vi "testoct.vi"() -> ()   [LabVIEW 2020]
uses:
  Utilities/Calculation related/Globals for GOLPI.vi
  external libraries/GOLPI 0.7.3.1 source distribution LV 20.0 32 bit/GOLPI library.lvlib
panel:
  in  "GNU Octave path":path
  out "error out":errorcluster
  in  "Stop":bool
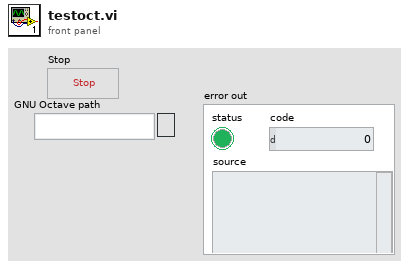
[diagram p1: front panel]
types:
  T1 = typedef "Type definitions to be saved.ctl" = cluster{"Common properties":T2, "AC Source":T3, "DC meter":T5, "CE measurement":T7, "FR measurement":T8, "FR template":T9, "CE template":T10, "PJVS":T11, "SS measurement":T15}
  T2 = typedef "Common properties.ctl" = cluster{"Measurement status ref":refnum<vi>, "TWM Status ref":refnum<vi>, "Abort ref":refnum<vi>, "Skip waiting ref":refnum<vi>, "GNU Octave path":path, "TWM+QWTB path":path, "lvlib path":path, "TWM pipe":string, "PJVS status ref":refnum<vi>, "WAC path":path}
  T3 = typedef "AC Source.ctl" = cluster{"AC Source type":T4, "VISA":refnum<visa-resource-name>, "Ref. clock (Hz)":dbl, "status ref":refnum<vi>}
  T4 = typedef "AC Source type.ctl" = enum16{"Fluke 5XXX calibrator", "Tektronix AFG3000 series", "dummy", "Agilent 331xxA to 332xxA", "Agilent 335xxA to 336xxA"}
  T5 = typedef "DC meter.ctl" = cluster{"DC meter type":T6, "DC meter VISA":refnum<visa-resource-name>, "NPLC":dbl, "status ref":refnum<vi>}
  T6 = typedef "DC meter type.ctl" = enum16{"H/A/K 3458", "Fluke 8508A", "dummy", "Keithley 2182"}
  T7 = typedef "CE measurement.ctl" = cluster{"Signal frequencies (Hz)":dbl[], "Signal amplitudes (V)":dbl[], "Sampling frequencies (Hz)":dbl[], "Record lengths (multiples of periods)":dbl[], "TWM data root directory":path, "TWM mreasurements directories":path[], "Calculate RMS from samples":bool, "RMS algorithm":string, "Settle down after AC source change (s)":dbl, "Skip PJVS setup":bool, "Measurement template file":path, "Row of START keyword":i32, "Row of STOP keyword":i32, "Measurement template line":i32[], "Switch position":dbl[], "FR fit mat file":path, "Recalculate-skip already calculated":bool}
  T8 = typedef "FR measuement.ctl" = cluster{"Measurement frequencies (Hz)":dbl[], "Sampling frequency (Hz)":dbl, "Signal amplitude (V)":dbl, "AC-DC settle time (s)":dbl, "Record length (multiples of period)":dbl[], "Measurement template file":path, "Row of START keyword":i32, "Row of STOP keyword":i32, "Calculate RMS from samples":bool, "AC-DC warm up time (s)":dbl, "Measurement template line":i32[], "DC meter readings No.":i32, "Algorithm":string, "Simultaneous measurement":bool, "Recalculate-skip already calculated":bool}
  T9 = typedef "FR template.ctl" = cluster{"Keywords column":i32, "Sig. freq. column":i32, "Rec. len. column":i32, "Meas. points. row min to read":i32, "Meas. points. row max to read":i32, "Properties column":i32, "Properties row start":i32, "Properties row end":i32, "Keyword START regexp":string, "Keyword STOP regexp":string, "HW data column":i32, "HW data row start":i32, "HW data row end":i32, "TIme and date column start":i32, "Digitizer value column start ":i32, "DC mean column start ":i32, "DC readings column start":i32}
  T10 = typedef "CE template.ctl" = cluster{"Keywords column":i32, "Sig. freq. column":i32, "Rec. len. column":i32, "Switch pos column":i32, "Meas. points. row min to read":i32, "Meas. points. row max to read":i32, "Properties column":i32, "Properties row start":i32, "Properties row end":i32, "Keyword START regexp":string, "Keyword STOP regexp":string, "HW data column":i32, "HW data row start":i32, "HW data row end":i32, "TIme and date column start":i32, "Digitizer value column start ":i32}
  T11 = typedef "PJVS.ctl" = cluster{"PJVS type":T12, "Status Refnum":refnum<vi>, "AC-supraVOLTcontrol":cluster{"IP address:port (0.0.0.0:0000)":string, "Timeouts":T13, "Simulation mode":bool, "Debug mode":bool}, "NPL bias source":cluster{"DataSocketCluster":T14}, "Manual PJVS":cluster{"PJVS frequency (Hz)":dbl, "Reference voltages (V)":dbl[], "File with PJVS voltages":path}, "VTT PJVS":cluster{"some VTT only property":string}}
  T12 = typedef "PJVS Type.ctl" = enum16{"AC-supraVOLTcontrol", "JV modified NPL bias control", "Manual PJVS", "VTT PJVS"}
  T13 = typedef "ACSVcontrol-driver.lvlib/Timeouts.ctl" = cluster{"TCP Read & Write (ms)":i32, "Sensors readout":i32, "PJVS setup":i32, "Nullmeter readout":i32, "Multiplexer setup":i32, "57XX setup":i32, "Generator setup":i32, "Synthesizer setup":i32, "Sampler readout":i32}
  T14 = typedef "DataSocketCluster external.ctl" = cluster{"Server Machine":string, "Client Machine":string, "Data":string, "TimeStamp":dbl, "Count":i32, "Target Process":string}
  T15 = typedef "SS measurement.ctl" = cluster{"Signal frequencies (Hz)":dbl[], "Signal amplitudes (V)":dbl[], "Sampling frequencies (Hz)":dbl[], "Record lengths (multiples of periods)":dbl[], "Calculate results":bool, "Algorithm":string, "TWM data directories":path[], "Settle down after AC source change (s)":dbl, "PJVS frequencies (Hz)":dbl[], "PJVS reference voltages":dbl[][], "Requested PJVS steps":u32[], "FR fit path":path, "Measure CE":bool, "Measure CE before":bool, "Measure CE after":bool, "CE fit path":path, "Measure digitizer gain":bool, "Measure digitizer gain before":bool, "Measure digitizer gain after":bool, "Digitizer gain":dbl}
  T16 = typedef "GOLPI library.lvlib/GOLPI reference Type Def.ctl" = cluster{"pipe handle":T17, "fast read timeout [ms]":u32, "fast read settle time [ms]":u32, "fast read to multiple [ms]":u32, "max elements per input line":u32, "slow read timeout [ms]":u32, "stdin double format specifier":string, "max elements per stdout output column":u32, "console mode bitstream":bool, "bitstream first read timeout [ms]":u32, "bitstream read timeout [ms]":u32, "struct transfer possible":bool, "matlab mode":bool}
  T17 = typedef "LV Process library.lvlib/Pipe Handle.ctl" = cluster{"lv_proc.dll file path":path, "process instance handle":u32[], "debug mode":bool, "debug data":cluster{"time":timestamp, "stdin":bool, "data":string}[]}
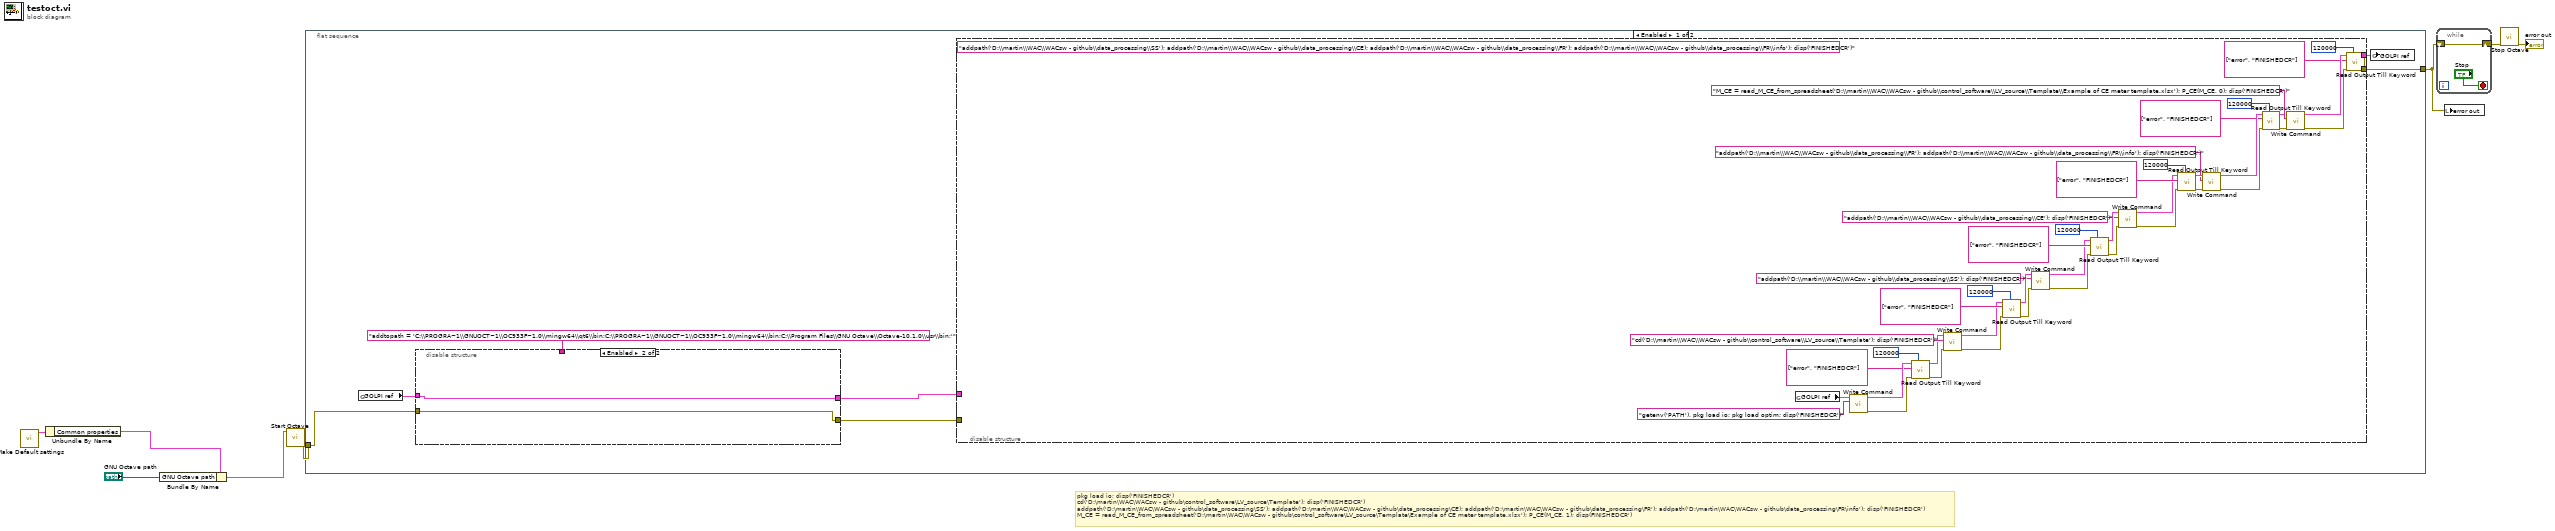
[diagram p0: block diagram]
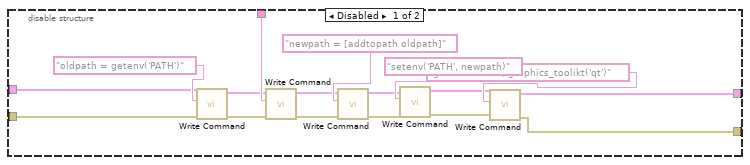
[diagram p2: hidden frame]
diagram:
  # "pkg load io; disp('FINISHEDCR')\ncd('D:\\martin\\WAC\\WACsw - github\\control_software\\LV_source\\Template'); disp('FINISHEDCR')\naddpath('D:\\martin\\WAC\\WACsw - github\\data_processing\\SS'); addpath('D:\\martin\\WAC\\WACsw - github\\data_processing\\CE); addpath('D:\\martin\\WAC\\WACsw - github\\data_processing\\FR'); addpath('D:\\martin\\WAC\\WACsw - github\\data_processing\\FR\\info'); disp('FINISHEDCR')\nM_CE = read_M_CE_from_spreadsheet('D:\\martin\\WAC\\WACsw - github\\control_software\\LV_source\\Template\\Example of CE meter template.xlsx'); P_CE(M_CE, 1); disp(FINISHEDCR')"
  n1 = call "Make Default settings.vi"() -> ("TD to be saved"=w6:T1)  [unwired: 11 in]
  n2 = Unbundle By Name(w6) -> ("Common properties"=w4:T2)
  n3 = Bundle By Name(cluster=w4, "GNU Octave path"="GNU Octave path") -> (w3:T2)
  n4 = call "Start Octave.vi"("Common properties"=w3) -> ("error out"=w5:errorcluster)  [unwired: 10 in]
  n5 = flat-sequence {
    tunnel: [w14] -> w1
    tunnel: w5 -> [w12]
    frame #0 {
      n6 = global read "Globals for GOLPI.vi" "GOLPI ref"() -> (w9:T16)
      n7 = disable-structure shown="Enabled" {
        disable-tunnel: "addtopath = 'C:\\PROGRA~1\\GNUOCT~1\\OC933F~1.0\\mingw64\\qt6\\bin;C:\\PROGRA~1\\GNUOCT~1\\OC933F~1.0\\mingw64\\bin;C:\\Program Files\\GNU Octave\\Octave-10.1.0\\usr\\bin;'" ("command") -> [w31 _]
        disable-tunnel: w12 -> [w19 w33]
        disable-tunnel: [w18 w33] -> w11
        disable-tunnel: [w17 w34] -> w10
        disable-tunnel: w9 -> [w16 w34]
        frame Disabled {
          n8 = call "Write Command.vi"("error in"=w19, "command"="oldpath = getenv('PATH')", "GOLPI ref. in"=w16) -> ("error out"=w27:errorcluster, "GOLPI ref. out"=w23:T16)  [unwired: 7 in]
          n9 = call "Write Command.vi"("error in"=w27, "command"=w31, "GOLPI ref. in"=w23) -> ("error out"=w26:errorcluster, "GOLPI ref. out"=w22:T16)  [unwired: 7 in]
          n10 = call "Write Command.vi"("error in"=w26, "command"="newpath = [addtopath oldpath]", "GOLPI ref. in"=w22) -> ("error out"=w25:errorcluster, "GOLPI ref. out"=w21:T16)  [unwired: 7 in]
          n11 = call "Write Command.vi"("error in"=w25, "command"="setenv('PATH', newpath)", "GOLPI ref. in"=w21) -> ("error out"=w24:errorcluster, "GOLPI ref. out"=w20:T16)  [unwired: 7 in]
          n12 = call "Write Command.vi"("error in"=w24, "command"="getenv('PATH'), graphics_toolikt('qt')", "GOLPI ref. in"=w20) -> ("error out"=w18:errorcluster, "GOLPI ref. out"=w17:T16)  [unwired: 7 in]
        }
        frame Enabled {
        }
      }
      n13 = disable-structure shown="Enabled" {
        disable-tunnel: [w53 w79] -> w15
        disable-tunnel: [w52 w78] -> w14
        disable-tunnel: w10 -> [_ w79]
        disable-tunnel: w11 -> [_ w78]
        frame Enabled {
          (unwired) "addpath('D:\\martin\\WAC\\WACsw - github\\data_processing\\SS'); addpath('D:\\martin\\WAC\\WACsw - github\\data_processing\\CE); addpath('D:\\martin\\WAC\\WACsw - github\\data_processing\\FR'); addpath('D:\\martin\\WAC\\WACsw - github\\data_processing\\FR\\info'); disp('FINISHEDCR')" ("command")
          n14 = global read "Globals for GOLPI.vi" "GOLPI ref"() -> (w54:T16)
          n15 = call "Write Command.vi"("command"="getenv('PATH'), pkg load io; pkg load optim; disp('FINISHEDCR')", "GOLPI ref. in"=w54) -> ("error out"=w77:errorcluster, "GOLPI ref. out"=w76:T16)  [unwired: 8 in]
          n16 = call "Read Output Till Keyword.vi"("timeout [ms]"=u32 120000, "error in"=w77, "keywords"=string[] ["error", "FINISHEDCR"], "GOLPI ref. in"=w76) -> ("error out"=w56:errorcluster, "GOLPI ref. out"=w55:T16)  [unwired: 4 in, 2 out]
          n17 = call "Write Command.vi"("error in"=w56, "command"="cd('D:\\martin\\WAC\\WACsw - github\\control_software\\LV_source\\Template'); disp('FINISHEDCR')", "GOLPI ref. in"=w55) -> ("error out"=w43:errorcluster, "GOLPI ref. out"=w42:T16)  [unwired: 7 in]
          n18 = call "Read Output Till Keyword.vi"("timeout [ms]"=u32 120000, "error in"=w43, "keywords"=string[] ["error", "FINISHEDCR"], "GOLPI ref. in"=w42) -> ("error out"=w45:errorcluster, "GOLPI ref. out"=w44:T16)  [unwired: 4 in, 2 out]
          n19 = call "Write Command.vi"("error in"=w45, "command"="addpath('D:\\martin\\WAC\\WACsw - github\\data_processing\\SS'); disp('FINISHEDCR')", "GOLPI ref. in"=w44) -> ("error out"=w41:errorcluster, "GOLPI ref. out"=w40:T16)  [unwired: 7 in]
          n20 = call "Read Output Till Keyword.vi"("timeout [ms]"=u32 120000, "error in"=w41, "keywords"=string[] ["error", "FINISHEDCR"], "GOLPI ref. in"=w40) -> ("error out"=w50:errorcluster, "GOLPI ref. out"=w51:T16)  [unwired: 4 in, 2 out]
          n21 = call "Write Command.vi"("error in"=w50, "command"="addpath('D:\\martin\\WAC\\WACsw - github\\data_processing\\CE'); disp('FINISHEDCR')", "GOLPI ref. in"=w51) -> ("error out"=w39:errorcluster, "GOLPI ref. out"=w38:T16)  [unwired: 7 in]
          n22 = call "Read Output Till Keyword.vi"("timeout [ms]"=u32 120000, "error in"=w39, "keywords"=string[] ["error", "FINISHEDCR"], "GOLPI ref. in"=w38) -> ("error out"=w58:errorcluster, "GOLPI ref. out"=w57:T16)  [unwired: 4 in, 2 out]
          n23 = call "Write Command.vi"("error in"=w58, "command"="addpath('D:\\martin\\WAC\\WACsw - github\\data_processing\\FR'); addpath('D:\\martin\\WAC\\WACsw - github\\data_processing\\FR\\info'); disp('FINISHEDCR')", "GOLPI ref. in"=w57) -> ("error out"=w71:errorcluster, "GOLPI ref. out"=w70:T16)  [unwired: 7 in]
          n24 = call "Read Output Till Keyword.vi"("timeout [ms]"=u32 120000, "error in"=w71, "keywords"=string[] ["error", "FINISHEDCR"], "GOLPI ref. in"=w70) -> ("error out"=w59:errorcluster, "GOLPI ref. out"=w60:T16)  [unwired: 4 in, 2 out]
          n25 = call "Write Command.vi"("error in"=w59, "command"="M_CE = read_M_CE_from_spreadsheet('D:\\martin\\WAC\\WACsw - github\\control_software\\LV_source\\Template\\Example of CE meter template.xlsx'); P_CE(M_CE, 0); disp('FINISHEDCR')", "GOLPI ref. in"=w60) -> ("error out"=w68:errorcluster, "GOLPI ref. out"=w69:T16)  [unwired: 7 in]
          n26 = call "Read Output Till Keyword.vi"("timeout [ms]"=u32 120000, "error in"=w68, "keywords"=string[] ["error", "FINISHEDCR"], "GOLPI ref. in"=w69) -> ("error out"=w52:errorcluster, "GOLPI ref. out"=w53:T16)  [unwired: 4 in, 2 out]
        }
        frame Disabled {
        }
      }
      n27 = global write "Globals for GOLPI.vi" "GOLPI ref"(w15) -> ()
    }
  }
  n28 = while {
    shift-right: [w80] -> w8
    shift-left: w1 -> [w80]
    stop <- "Stop" stop-if-true
  }
  n29 = local write "error out"(w1) -> ()
  n30 = call "Stop Octave.vi"("error in (no error)"=w8) -> ("error out"=→"error out":errorcluster)  [unwired: 10 in]
